vi "Initialize.vi"(8 "error in (no error)":errorcluster, 11 "Bronkhorst Settings in":T1={"VISA resource name"="", "Simulated?"=FALSE, "Smoothing Steps"=1} {"Smoothing Steps" min=1 step=1}) -> (0 "error out":errorcluster, 2 "No Meter Connnected":bool, 3 "Bronkhorst Settings out":T1={"VISA resource name"="", "Simulated?"=FALSE, "Smoothing Steps"=1} {"Smoothing Steps" min=1 step=1})   [LabVIEW 2018, in "Bronkhorst M13 Flow Meter.lvlib"]
uses:
  Bronkhorst M13 Flow Meter.lvlib
  Settings Cluster.ctl
  <vilib>/Instr/_visa.llb/VISA Configure Serial Port (Instr).vi
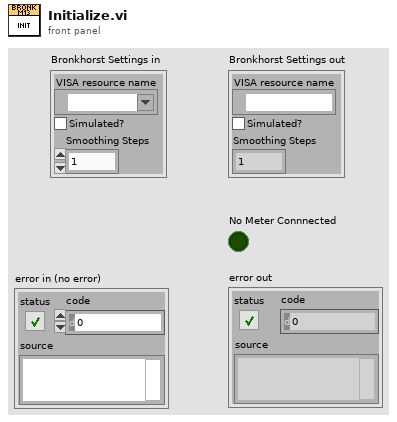
[diagram p1: front panel]
types:
  T1 = typedef "Bronkhorst M13 Flow Meter.lvlib/Settings Cluster.ctl" = cluster{"VISA resource name":refnum<visa-resource-name>, "Simulated?":bool, "Smoothing Steps":i32}
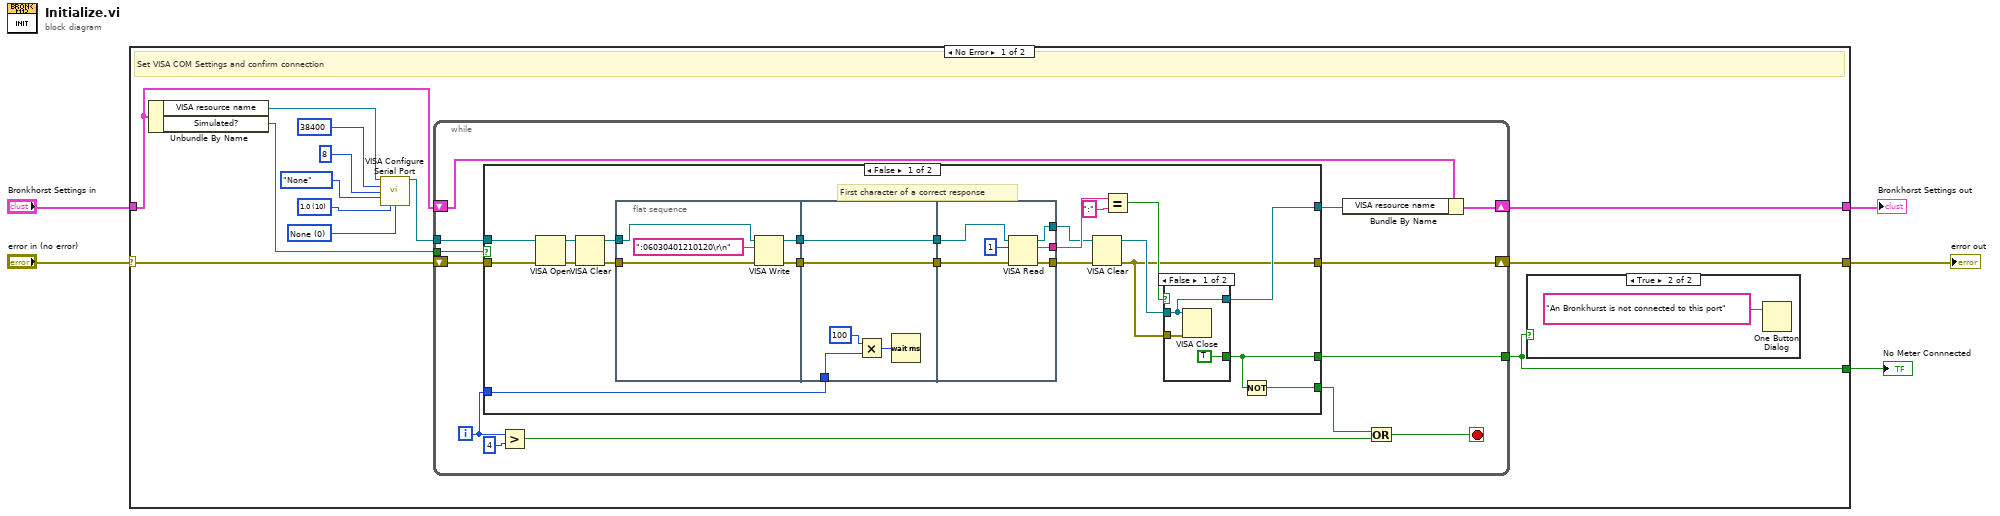
[diagram p0: block diagram]
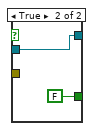
[diagram p3: hidden frame]
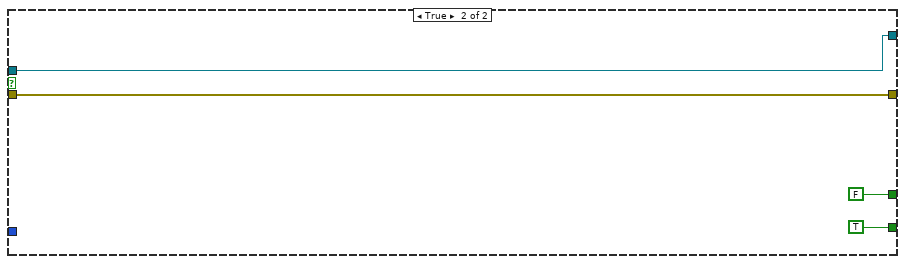
[diagram p4: hidden frame]
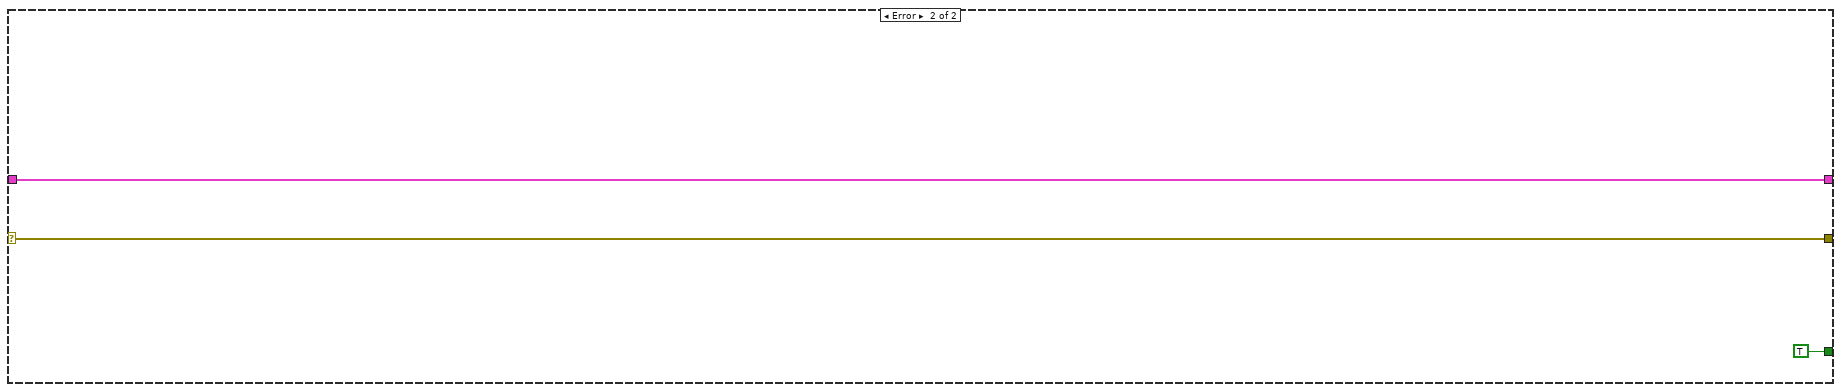
[diagram p5: hidden frame]
diagram:
  n1 = case shown="No Error" "error in (no error)" {
    selector: "error in (no error)" -> [w18 w81]
    tunnel: "Bronkhorst Settings in" -> [w16 w80]
    tunnel: [w14 w81] -> w4
    tunnel: [w15 w80] -> w2
    tunnel: [w13 TRUE] -> w1
    frame No Error {
      w8 = u16 0 items=["None", "XON/XOFF", "RTS/CTS", "XON/XOFF & RTS/CTS", "DTR/DSR", "XON/XOFF & DTR/DSR"] ("flow control (0:none)")
      w9 = u16 10 items=["1.0"=10, "1.5"=15, "2.0"=20] ("stop bits (10: 1 bit)")
      # "Set VISA COM Settings and confirm connection"
      n2 = Unbundle By Name(w16) -> ("VISA resource name"=w7:refnum<visa-resource-name>, "Simulated?"=w17:bool)
      n3 = call-poly "VISA Configure Serial Port"("VISA resource name"=w7, "baud rate (9600)"=u32 38400, "data bits (8)"=u16 8, "parity (0:none)"=enum16{"None", "Odd", "Even", "Mark", "Space"}."None", "stop bits (10: 1 bit)"=w9, "flow control (0:none)"=w8) -> ("VISA resource name out"=w6:refnum<visa-resource-name>)  [unwired: 8 in, 1 out]
      n4 = while {
        tunnel: w17 -> [w31]
        shift-right: [w27] -> w14
        shift-left: w18 -> [w32]
        shift-right: [w29] -> w15
        shift-left: w16 -> [w30]
        tunnel: [w21] -> w13
        tunnel: w6 -> [w20]
        i -> [w26]
        stop <- w25 stop-if-true
        n5 = case shown="False" w31 {
          tunnel: w32 -> [w34 w78]
          tunnel: [w33 w78] -> w27
          tunnel: w20 -> [w35 w77]
          tunnel: [w42 w77] -> w28
          tunnel: [w38 TRUE] -> w23
          tunnel: w26 -> [w37 _]
          tunnel: [w36 FALSE] -> w21
          frame False {
            # "First character of a correct response"
            n6 = VISA Open(error in (no error)=w34, VISA resource name=w35) -> (VISA resource name=w39:refnum<visa-resource-name>, error out=w53:errorcluster)  [unwired: 3 in]
            n7 = VISA Clear(VISA resource name=w39, error in (no error)=w53) -> (VISA resource name out=w40:refnum<visa-resource-name>, error out=w41:errorcluster)
            n8 = flat-sequence {
              tunnel: w41 -> [w58]
              tunnel: [w56] -> w52
              tunnel: [w55] -> w51
              tunnel: w40 -> [w54]
              tunnel: w52 -> [w63]
              tunnel: [w63] -> w50
              tunnel: w51 -> [w62]
              tunnel: [w62] -> w49
              tunnel: w37 -> [w60]
              tunnel: [w69] -> w44
              tunnel: [w68] -> w47
              tunnel: [w67] -> w43
              tunnel: w50 -> [w66]
              tunnel: w49 -> [w65]
              frame #0 {
                n9 = VISA Write(VISA resource name=w54, write buffer=":06030401210120\r\n", error in (no error)=w58) -> (VISA resource name out=w56:refnum<visa-resource-name>, error out=w55:errorcluster)  [unwired: 1 out]
              }
              frame #1 {
                n10 = Multiply(x=u32 100 ("milliseconds to wait"), y=w60) -> (x*y=w59:u32)
                n11 = Wait (ms)(milliseconds to wait=w59) -> ()  [unwired: 1 out]
              }
              frame #2 {
                n12 = VISA Read(VISA resource name=w66, byte count=u32 1, error in (no error)=w65) -> (VISA resource name out=w67:refnum<visa-resource-name>, read buffer=w68:string, error out=w69:errorcluster)  [unwired: 1 out]
              }
            }
            n13 = VISA Clear(VISA resource name=w43, error in (no error)=w44) -> (VISA resource name out=w45:refnum<visa-resource-name>, error out=w33:errorcluster)
            n14 = Equal?(x=w47, y=":") -> (x = y?=w48:bool)
            n15 = case shown="False" w48 {
              tunnel: w45 -> [w71 w74]
              tunnel: w33 -> [w72 _]
              tunnel: [w71 w74] -> w42
              tunnel: [TRUE FALSE] -> w36
              frame False {
                n16 = VISA Close(VISA resource name=w71, error in (no error)=w72) -> ()  [unwired: 1 out]
              }
              frame True {
              }
            }
            n17 = Not(x=w36) -> (.not. x?=w38:bool)
          }
          frame True {
          }
        }
        n18 = Greater?(x=w26, y=4) -> (0:w24:bool)
        n19 = Bundle By Name(cluster=w30, "VISA resource name"=w28) -> (w29:T1)
        n20 = Or(x=w23, y=w24) -> (x .or. y?=w25:bool)
      }
      n21 = case shown="True" w13 {
        frame False {
        }
        frame True {
          n22 = One Button Dialog(message="An Bronkhurst is not connected to this port") -> ()  [unwired: 1 in, 1 out]
        }
      }
    }
    frame Error {
    }
  }
  "error out" <- w4
  "Bronkhorst Settings out" <- w2
  "No Meter Connnected" <- w1
